vi "Cryomagnetics Get Sweep Mode.vi"(8 "error in (no error)":errorcluster, 11 "VISA Resource Name":refnum<visa-resource-name>) -> (0 "error out":errorcluster, 2 "sweep mode":T1, 3 "VISA Resource Name Out":refnum<visa-resource-name>)   [LabVIEW 2015]
uses:
  Sweep mode.ctl
  GPIB/VISA  Send Receive.vi
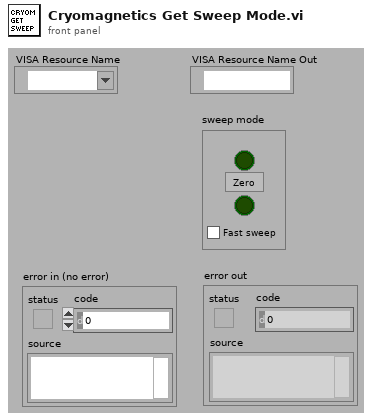
[diagram p1: front panel]
types:
  T1 = typedef "Sweep mode.ctl" = cluster{"zero":bool, "sweep up":bool, "sweep down":bool, "fast sweep":bool}
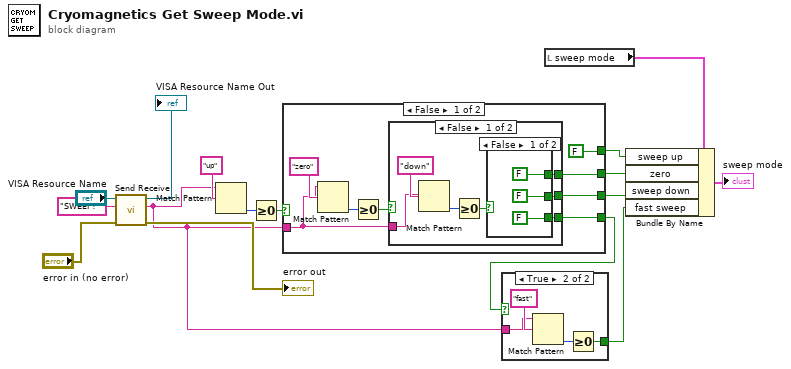
[diagram p0: block diagram]
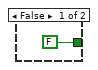
[diagram p2: hidden frame]
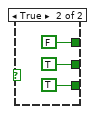
[diagram p3: hidden frame]
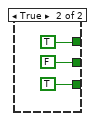
[diagram p4: hidden frame]
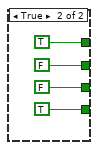
[diagram p5: hidden frame]
diagram:
  n1 = call-poly "Send Receive.vi"("error in (no error)"="error in (no error)", "data string in"="SWEEP?", "VISA Resource Name"="VISA Resource Name") -> ("error out"=→"error out":errorcluster, "data string out"=w1:string, "VISA Resource Name Out"=→"VISA Resource Name Out":refnum<visa-resource-name>)  [unwired: 6 in]
  n2 = Match Pattern(string=w1, regular expression="up") -> (offset past match=w16:i32)  [unwired: 1 in, 3 out]
  n3 = Greater Or Equal To 0?(x=w16) -> (x >= 0?=w15:bool)
  n4 = case shown="False" w15 {
    tunnel: w1 -> [w21 _]
    tunnel: [w20 FALSE] -> w12
    tunnel: [w19 TRUE] -> w13
    tunnel: [w18 FALSE] -> w11
    tunnel: [FALSE TRUE] -> w10
    frame False {
      n5 = Match Pattern(string=w21, regular expression="zero") -> (offset past match=w24:i32)  [unwired: 1 in, 3 out]
      n6 = Greater Or Equal To 0?(x=w24) -> (x >= 0?=w22:bool)
      n7 = case shown="False" w22 {
        tunnel: w21 -> [w29 _]
        tunnel: [w26 FALSE] -> w20
        tunnel: [w25 TRUE] -> w19
        tunnel: [w27 TRUE] -> w18
        frame False {
          n8 = Match Pattern(string=w29, regular expression="down") -> (offset past match=w30:i32)  [unwired: 1 in, 3 out]
          n9 = Greater Or Equal To 0?(x=w30) -> (x >= 0?=w28:bool)
          n10 = case shown="False" w28 {
            tunnel: [FALSE FALSE] -> w27
            tunnel: [FALSE TRUE] -> w26
            tunnel: [FALSE TRUE] -> w25
            frame False {
            }
            frame True {
            }
          }
        }
        frame True {
        }
      }
    }
    frame True {
    }
  }
  n11 = case shown="True" w13 {
    tunnel: w1 -> [_ w47]
    tunnel: [FALSE w46] -> w9
    frame False {
    }
    frame True {
      n12 = Match Pattern(string=w47, regular expression="fast") -> (offset past match=w48:i32)  [unwired: 1 in, 3 out]
      n13 = Greater Or Equal To 0?(x=w48) -> (x >= 0?=w46:bool)
    }
  }
  n14 = local read "sweep mode"() -> (w7:T1)
  n15 = Bundle By Name(cluster=w7, "sweep up"=w10, "zero"=w11, "sweep down"=w12, "fast sweep"=w9) -> (→"sweep mode":T1)
